vi "Append to report.vi"(8 "error in (no error)":errorcluster, 9 "Value":string, 10 "Key":string, 11 "Plain Text Report In":refnum<class "Plain Text Report.lvclass">) -> (0 "error out":errorcluster, 3 "Plain Text Report Out":refnum<class "Plain Text Report.lvclass">)   [LabVIEW 2020, in "Plain Text Report.lvclass"]
uses:
  Plain Text Report.lvclass
  Plain Text Report.lvclass/Plain Text Report.ctl
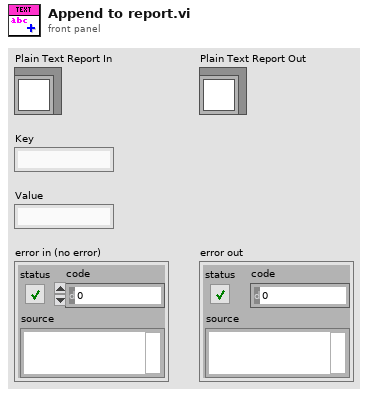
[diagram p1: front panel]
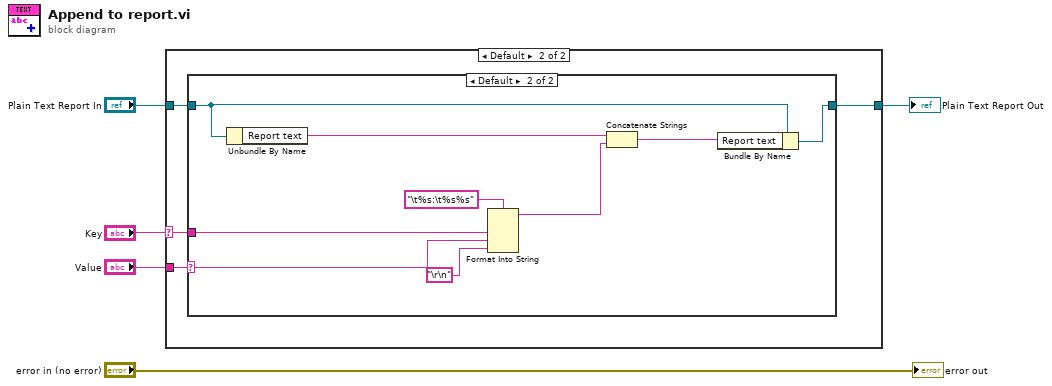
[diagram p0: block diagram]
diagram:
  n1 = case shown="Default" "Key" {
    selector: "Key" -> [_ w9]
    tunnel: "Plain Text Report In" -> [w6 w10]
    tunnel: "Value" -> [_ w8]
    tunnel: [w6 w7] -> w2
    frame "" {
    }
    frame Default {
      n2 = case shown="Default" w8 {
        selector: w8 -> [_ w17]
        tunnel: w10 -> [w11 w20]
        tunnel: w9 -> [_ w18]
        tunnel: [w11 w15] -> w7
        frame "" {
        }
        frame Default {
          n3 = Unbundle By Name(w20) -> ("Report text"=w19:string)
          n4 = Format Into String(format string="\t%s:\t%s%s", w18, w17, "\r\n") -> (resulting string=w16:string)  [unwired: 2 in, 1 out]
          n5 = Concatenate Strings(w19, w16) -> (w14:string)
          n6 = Bundle By Name(cluster=w20, "Report text"=w14) -> (w15:refnum<class "Plain Text Report.lvclass">)
        }
      }
    }
  }
  "Plain Text Report Out" <- w2
  "error out" <- "error in (no error)"
